vi "Setup subWorker - sequenceManagerWkr.vi"(8 "error in":errorcluster, 11 "sequenceManagerTest in":refnum<class "sequenceManagerTest.lvclass">) -> (0 "error out":errorcluster, 3 "sequenceManagerTest out":refnum<class "sequenceManagerTest.lvclass">)   [LabVIEW 2023, in "sequenceManagerTest.lvclass"]
doc: "This VI sets up the framework parameters of a statically-linked subWorker."
uses:
  sequenceManagerTest.lvclass
  sequenceManagerTest.lvclass/sequenceManagerTest.ctl
  sequenceManagerWorker/sequenceManagerWorker.lvclass
  C:/Program Files (x86)/National Instruments/LabVIEW 2023/vi.lib/addons/_Workers/Library/Classes/Worker/Worker.lvclass
  C:/Program Files (x86)/National Instruments/LabVIEW 2023/vi.lib/addons/_Workers/Library/Classes/Workers Object/Workers Object.lvclass
  C:/Cutiss/ZE_Easy.SequenceManager/LabViewWrapper/Easy.SequenceManager.Worker/Workers/sequenceManagerWorker/sequenceManagerWorker.lvclass
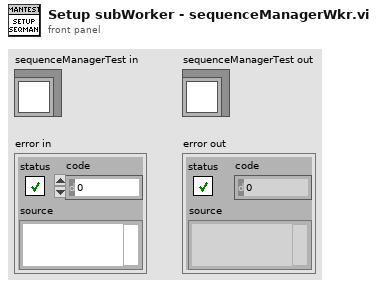
[diagram p1: front panel]
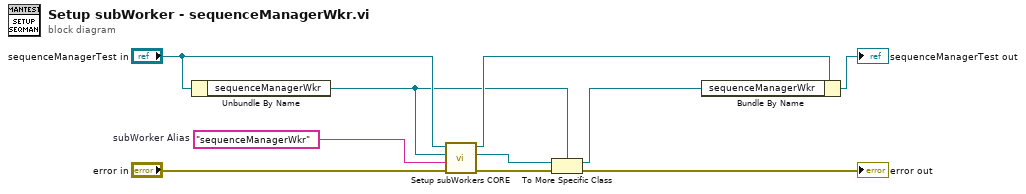
[diagram p0: block diagram]
diagram:
  w6 = "sequenceManagerWkr"  # subWorker Alias
  n1 = Unbundle By Name("sequenceManagerTest in") -> ("sequenceManagerWkr"=w3:refnum<class "sequenceManagerWorker.lvclass">)
  n2 = call-dynamic "Setup subWorkers CORE.vi"("error in"="error in", "subWorker Alias"=w6, "subWorker"=w3, "Worker"="sequenceManagerTest in") -> ("error out"=w5:errorcluster, "subWorker out"=w1:refnum<class "Worker.lvclass">, "Worker out"=w8:refnum<class "sequenceManagerTest.lvclass">)  [unwired: 5 in]
  n3 = To More Specific Class(target class=w3, reference=w1, error in=w5) -> (specific class reference=w2:refnum<class "sequenceManagerWorker.lvclass">, error out=→"error out":errorcluster)
  n4 = Bundle By Name(cluster=w8, "sequenceManagerWkr"=w2) -> (→"sequenceManagerTest out":refnum<class "sequenceManagerTest.lvclass">)
